vi "FPGAController_v6_Debug.vi"() -> ()   [LabVIEW 2015]
uses:
  Limits_In.ctl
  <vilib>/Utility/miscctls.llb/LVPointTypeDef.ctl
  <vilib>/FPGAPlugInAG/PXIe-7971R/niLvFpga_Open_PXIe-7971R.vi
  <vilib>/Utility/error.llb/Error Cluster From Error Code.vi
  <vilib>/rvi/errors/niLvFpgaAdjustHostInterfaceError.vi
  <userlib>/_OpenG.lib/comparison/comparison.llb/Variant Changed__ogtk.vi
  <vilib>/FPGAPlugInAG/PXIe-7971R/niLvFpga_Close_PXIe-7971R.vi
  <vilib>/rvi/interface/nirviOpenFPGA/nirviOpenFPGA.xnode
  FPGA Bitfiles/FPGA3_FPGATarget_FPGAcode4Test_4n9bj2mwd9A.lvbitx
  <vilib>/rvi/interface/nirviReadWriteControl/nirviReadWriteControl.xnode
  <vilib>/rvi/interface/nirviCloseFPGA/nirviCloseFPGA.xnode
  NiFpgaLv.dll
panel:
  in  "stop":bool
  in  "Tab Control":T1(tab)
  in  "User Trigger?":bool
  in  "User Trigger Distance":fxp<+/-,34,18> format="%.3g"
  in  "Arm/Disarm PSU":bool
  in  "One Shot":bool
  in  "Calibrate":bool
  in  "Threshold Factor":fxp<+/-,32,16>=1.0 format="%.2g"
  out "Limits":T2
  out "Armed":bool
  in  "Clear Points":bool
  in  "Calibration Time (ms)":u32=500
  in  "Boxcar 3 Size Factor":fxp<+/-,32,16>=0.1999969482421875 format="%.2g"
  in  "Charge Error Factor":fxp<+/-,32,16>=1.100006103515625 format="%.2g"
  in  "Max Correlation Factor":fxp<+,32,4>=0.25 format="%.3g"
  out "Latest Particle Stats":T3
  out "Discard Points":i32[][](graph)
  in  "error in (no error)":errorcluster
  out "error out":errorcluster
  out "Runtime Error":errorcluster
  # "User Trigger Distance is\nmeasured in meters from the\nend of the LEIL Chamber\nclosest to the Third Detector"
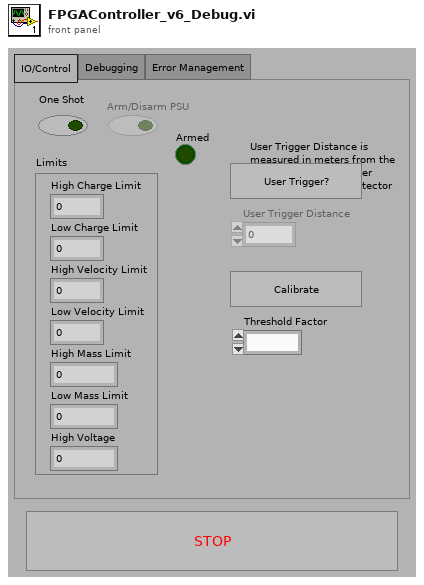
[diagram p1: front panel]
types:
  T1 = enum32{"IO/Control", "Debugging", "Error Management"}
  T2 = typedef "Limits_In.ctl" = cluster{"High Charge Limit":fxp<+,32,-41>, "Low Charge Limit":fxp<+,32,-41>, "High Velocity Limit":fxp<+,18,18>, "Low Velocity Limit":fxp<+,18,18>, "High Mass Limit":fxp<+/-,33,-35>, "Low Mass Limit":fxp<+/-,33,-35>, "High Voltage":fxp<+,16,22>}
  T3 = cluster{"Charge":dbl, "Mass":dbl, "Velocity":i32}
  T4 = enum8{"Enabled", "Disabled", "Disabled and Grayed Out"}
  T5 = typedef "LVPointTypeDef.ctl" = cluster{"Horizontal":i16, "Vertical":i16}
  T6 = cluster{"[0]":fxp<+/-,64,-10>, "[1]":fxp<+/-,64,-10>, "[2]":fxp<+/-,64,-10>, "[3]":fxp<+/-,64,-10>, "[4]":fxp<+/-,64,-10>, "[5]":fxp<+/-,64,-10>, "[6]":fxp<+/-,64,-10>, "[7]":fxp<+/-,64,-10>, "[8]":fxp<+/-,64,-10>, "[9]":fxp<+/-,64,-10>, "[10]":fxp<+/-,64,-10>}
  T7 = cluster{"[0]":fxp<+/-,64,-2>, "[1]":fxp<+/-,64,-2>, "[2]":fxp<+/-,64,-2>, "[3]":fxp<+/-,64,-2>, "[4]":fxp<+/-,64,-2>, "[5]":fxp<+/-,64,-2>, "[6]":fxp<+/-,64,-2>, "[7]":fxp<+/-,64,-2>, "[8]":fxp<+/-,64,-2>, "[9]":fxp<+/-,64,-2>, "[10]":fxp<+/-,64,-2>}
  T8 = cluster{"[0]":i32, "[1]":i32, "[2]":i32, "[3]":i32, "[4]":i32, "[5]":i32, "[6]":i32, "[7]":i32, "[8]":i32, "[9]":i32, "[10]":i32}
  T9 = cluster{"Discard Points 1":cluster{"1":i32, "2":i32, "3":i32, "4":i32, "5":i32, "6":i32, "7":i32, "8":i32, "9":i32, "10":i32, "11":i32}, "Discard Points 2":cluster{"1":i32, "2":i32, "3":i32, "4":i32, "5":i32, "6":i32, "7":i32, "8":i32, "9":i32, "10":i32, "11":i32}, "Discard Points 3":cluster{"1":i32, "2":i32, "3":i32, "4":i32, "5":i32, "6":i32, "7":i32, "8":i32, "9":i32, "10":i32, "11":i32}, "Discard Points 4":cluster{"1":i32, "2":i32, "3":i32, "4":i32, "5":i32, "6":i32, "7":i32, "8":i32, "9":i32, "10":i32, "11":i32}, "Discard Points 5":cluster{"1":i32, "2":i32, "3":i32, "4":i32, "5":i32, "6":i32, "7":i32, "8":i32, "9":i32, "10":i32, "11":i32}, "Discard Points 6":cluster{"1":i32, "2":i32, "3":i32, "4":i32, "5":i32, "6":i32, "7":i32, "8":i32, "9":i32, "10":i32, "11":i32}, "Discard Points 7":cluster{"1":i32, "2":i32, "3":i32, "4":i32, "5":i32, "6":i32, "7":i32, "8":i32, "9":i32, "10":i32, "11":i32}, "Discard Points 8":cluster{"1":i32, "2":i32, "3":i32, "4":i32, "5":i32, "6":i32, "7":i32, "8":i32, "9":i32, "10":i32, "11":i32}, "Discard Points 9":cluster{"1":i32, "2":i32, "3":i32, "4":i32, "5":i32, "6":i32, "7":i32, "8":i32, "9":i32, "10":i32, "11":i32}, "Discard Points 10":cluster{"1":i32, "2":i32, "3":i32, "4":i32, "5":i32, "6":i32, "7":i32, "8":i32, "9":i32, "10":i32, "11":i32}, "Discard Points 11":cluster{"1":i32, "2":i32, "3":i32, "4":i32, "5":i32, "6":i32, "7":i32, "8":i32, "9":i32, "10":i32, "11":i32}}
  T10 = cluster{"1":i32, "2":i32, "3":i32, "4":i32, "5":i32, "6":i32, "7":i32, "8":i32, "9":i32, "10":i32, "11":i32}[]
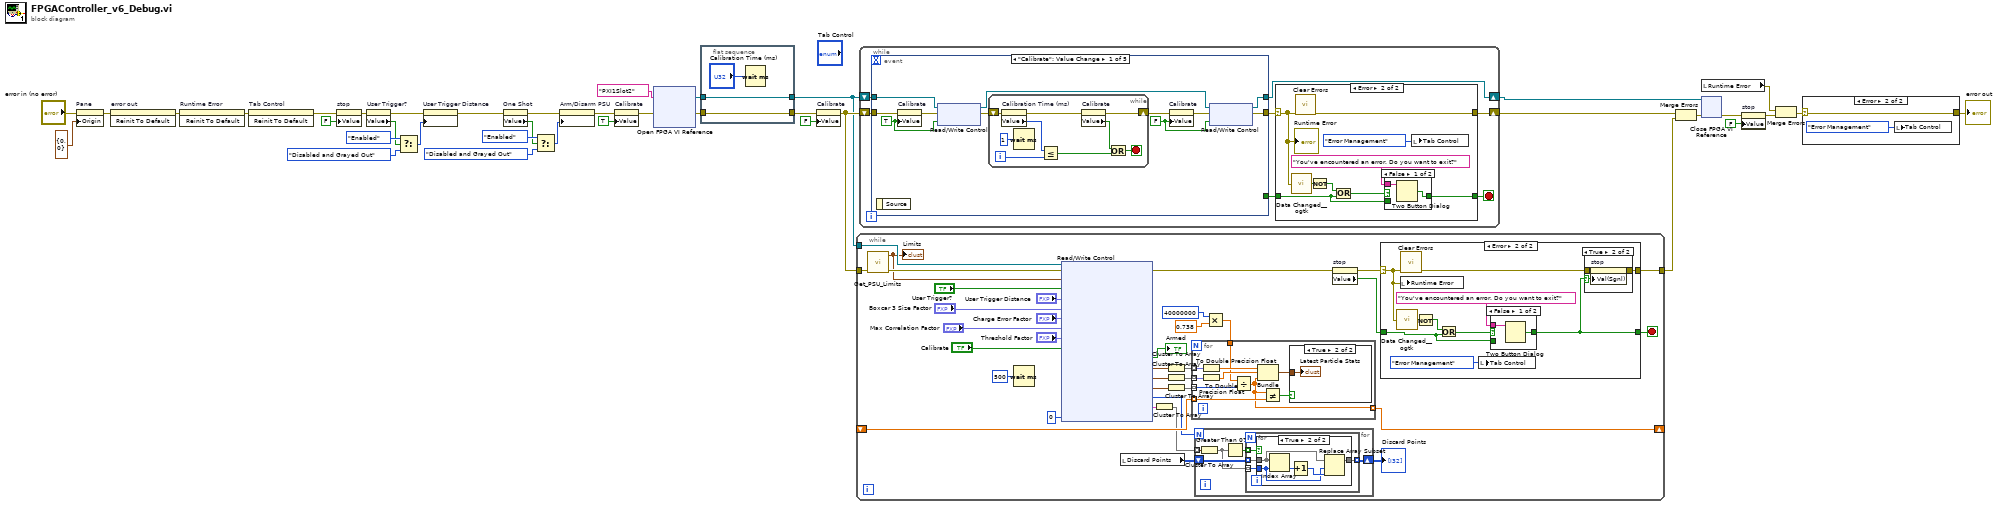
[diagram p0: block diagram]
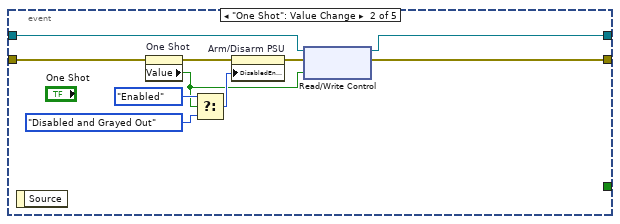
[diagram p10: hidden frame]
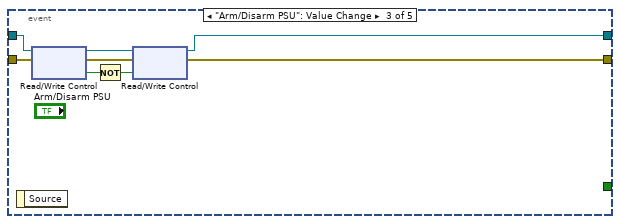
[diagram p11: hidden frame]
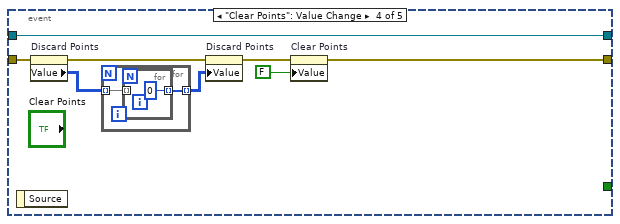
[diagram p12: hidden frame]
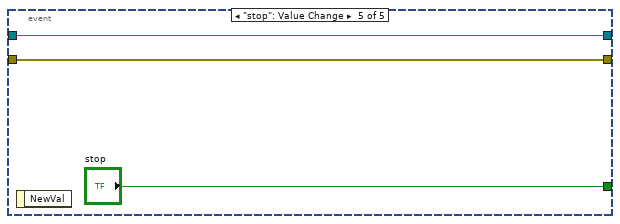
[diagram p13: hidden frame]
diagram:
  n1 = property on="Pane" class="Pane"(error in="error in (no error)", "Origin"=T5 {"Horizontal"=0, "Vertical"=0}) -> (error out=w17:errorcluster)  [unwired: 1 in, 1 out]
  n2 = invoke on="error out" class="Clust (strict)" method="Reinit To Default"(error in=w17) -> (error out=w18:errorcluster)  [unwired: 2 in, 2 out]
  n3 = invoke on="Runtime Error" class="Clust (strict)" method="Reinit To Default"(error in=w18) -> (error out=w16:errorcluster)  [unwired: 2 in, 2 out]
  n4 = invoke on="Tab Control" class="TabCtl (strict)" method="Reinit To Default"(error in=w16) -> (error out=w15:errorcluster)  [unwired: 2 in, 2 out]
  n5 = property on="stop" class="Bool (strict)"(error in=w15, "Value"=FALSE ("stop")) -> (error out=w10:errorcluster)  [unwired: 1 in, 1 out]
  n6 = property on="User Trigger?" class="Bool (strict)"(error in=w10) -> (error out=w20:errorcluster, "Value"=w11:bool)  [unwired: 1 in, 1 out]
  n7 = Select(t=T4."Enabled" ("Disabled"), s=w11, f=T4."Disabled and Grayed Out" ("Disabled")) -> (s? t:f=w22:T4)
  n8 = property on="User Trigger Distance" class="DigNum (strict)"(error in=w20, "DisabledEnum"=w22) -> (error out=w9:errorcluster)  [unwired: 1 in, 1 out]
  n9 = property on="One Shot" class="Bool (strict)"(error in=w9) -> (error out=w29:errorcluster, "Value"=w12:bool)  [unwired: 1 in, 1 out]
  n10 = Select(t=T4."Enabled" ("Disabled"), s=w12, f=T4."Disabled and Grayed Out" ("Disabled")) -> (s? t:f=w23:T4)
  n11 = property on="Arm/Disarm PSU" class="Bool"(error in=w29, "DisabledEnum"=w23) -> (error out=w8:errorcluster)  [unwired: 1 in, 1 out]
  n12 = property on="Calibrate" class="Bool (strict)"(error in=w8, "Value"=TRUE ("One Shot")) -> (error out=w13:errorcluster)  [unwired: 1 in, 1 out]
  n13 = xnode "Open FPGA VI Reference"("error in"=w13, "resource name"=tag "PXI1Slot2") -> ("FPGA VI Reference Out"=w27:refnum<k20>, "error out"=w1:errorcluster)
  n14 = flat-sequence {
    tunnel: [w41] -> w3
    tunnel: w27 -> [w41]
    tunnel: [w40] -> w2
    tunnel: w1 -> [w40]
    frame #0 {
      n15 = Wait (ms)(milliseconds to wait="Calibration Time (ms)") -> ()  [unwired: 1 out]
    }
  }
  n16 = property on="Calibrate" class="Bool (strict)"(error in=w2, "Value"=FALSE ("One Shot")) -> (error out=w6:errorcluster)  [unwired: 1 in, 1 out]
  n17 = while {
    tunnel: [w74] -> w4
    tunnel: w6 -> [w72]
    tunnel: w3 -> [w73]
    shift-right: [w54] -> _
    shift-left: _ -> [w53]
    stop <- w77 stop-if-true
    n18 = call "Get_PSU_Limits.vi"("error in (no error)"=w72) -> ("error out"=w71:errorcluster, "Limits"=w70:T2)  [unwired: 9 in]
    "Limits" <- w70
    n19 = Wait (ms)(milliseconds to wait=u32 500) -> ()  [unwired: 1 out]
    n20 = xnode "Read/Write Control"("FPGA VI Reference In"=w73, "error in"=w71, "Limits"=w70, "User Trigger?"="User Trigger?", "User Trigger Distance"="User Trigger Distance", "Boxcar 3 Size Factor"="Boxcar 3 Size Factor", "Charge Error Factor"="Charge Error Factor", "Max Correlation Factor"="Max Correlation Factor", "Threshold Factor"="Threshold Factor", "Calibrate"="Calibrate", "Particles Discarded"=i16 0) -> ("error out"=w47:errorcluster, "Armed"=→"Armed":bool, "Charge"=w60:T6, "Mass"=w59:T7, "Velocity Count"=w58:T8, "Particles Discarded"=w52:i16, "All Discard Points"=w44:T9)  [unwired: 1 out]
    n21 = local read "Discard Points"() -> (w46:i32[][])
    n22 = Cluster To Array(cluster=w44) -> (array=w51:T10)
    n23 = Cluster To Array(cluster=w60) -> (array=w57:fxp<+/-,64,-10>[])
    n24 = Cluster To Array(cluster=w59) -> (array=w56:fxp<+/-,64,-2>[])
    n25 = Cluster To Array(cluster=w58) -> (array=w55:i32[])
    n26 = for {
      N: w52 -> [_]
      tunnel: w51 -> [w82] mode=indexing
      shift-right: [w78] -> w45
      shift-left: w46 -> [w81]
      n27 = Cluster To Array(cluster=w82) -> (array=w79:i32[])
      n28 = Greater Than 0?(x=w79) -> (x > 0?=w80:bool[])
      n29 = for {
        tunnel: w81 -> [w86] mode=indexing
        tunnel: w79 -> [w85] mode=indexing
        tunnel: w80 -> [w84] mode=indexing
        tunnel: [w83] -> w78 mode=indexing
        n30 = case shown="True" w84 {
          tunnel: w86 -> [w87 w90]
          tunnel: w85 -> [_ w89]
          tunnel: [w87 w88] -> w83
          frame False {
          }
          frame True {
            n31 = Index Array(array=w90, index=w89) -> (element=w92:i32)
            n32 = Increment(x=w92) -> (x+1=w91:i32)
            n33 = Replace Array Subset(array=w90, new element=w91, index=w89) -> (w88:i32[])
          }
        }
      }
    }
    "Discard Points" <- w45
    n34 = Multiply(x=40000000, y=0.738) -> (x*y=w48:dbl)
    n35 = for {
      tunnel: w57 -> [w102] mode=indexing
      tunnel: w56 -> [w101] mode=indexing
      tunnel: w55 -> [w95] mode=indexing
      tunnel: [w93] -> w54 mode=indexing
      tunnel: w53 -> [w94] mode=indexing
      tunnel: w48 -> [w96]
      n36 = To Double Precision Float(number=w102) -> (double precision float=w100:dbl)
      n37 = To Double Precision Float(number=w101) -> (double precision float=w99:dbl)
      n38 = Divide(x=w96, y=w95) -> (x/y=w93:dbl)
      n39 = Bundle(w100, w99, w93) -> (w97:cluster{dbl, dbl, dbl})  [unwired: 1 in]
      n40 = Not Equal?(x=w93, y=w94) -> (x != y?=w98:bool)
      n41 = case shown="True" w98 {
        tunnel: w97 -> [_ w103]
        frame False {
        }
        frame True {
          "Latest Particle Stats" <- w103
        }
      }
    }
    n42 = property on="stop" class="Bool (strict)"(error in=w47) -> (error out=w76:errorcluster, "Value"=w75:bool)  [unwired: 1 in, 1 out]
    n43 = case shown="Error" w76 {
      selector: w76 -> [w105 w110]
      tunnel: [w105 w109] -> w74
      tunnel: [w104 w107] -> w77
      tunnel: w75 -> [w104 w111]
      frame No Error {
      }
      frame Error {
        n44 = call-poly <userlib>:"Data Changed__ogtk.vi"("Variant"=w110) -> ("Changed"=w113:bool)
        n45 = local write "Runtime Error"(w110) -> ()
        n46 = call <vilib>:"Clear Errors.vi"("error in (no error)"=w110) -> ("error out"=w108:errorcluster)  [unwired: 5 in, 1 out]
        n47 = Not(x=w113) -> (.not. x?=w112:bool)
        n48 = Or(x=w112, y=w111) -> (x .or. y?=w114:bool)
        n49 = local write "Tab Control"(T1."Error Management" ("Tab Control")) -> ()
        n50 = case shown="False" w114 {
          tunnel: "You've encountered an error. Do you want to exit?" ("message") -> [w121 _]
          tunnel: [w120 w122] -> w107
          tunnel: w111 -> [_ w122]
          frame False {
            n51 = Two Button Dialog(message=w121) -> (T button?=w120:bool)  [unwired: 2 in]
          }
          frame True {
          }
        }
        n52 = case shown="True" w107 {
          selector: w107 -> [_ w117]
          tunnel: [w116 w119] -> w109
          tunnel: w108 -> [w116 w118]
          frame False {
          }
          frame True {
            n53 = property on="stop" class="Bool (strict)"(error in=w118, "Val(Sgnl)"=w117) -> (error out=w119:errorcluster)  [unwired: 1 in, 1 out]
          }
        }
      }
    }
  }
  n54 = while {
    shift-right: [w123] -> w36
    shift-left: w6 -> [w129]
    shift-right: [w127] -> w37
    shift-left: w3 -> [w128]
    stop <- w125 stop-if-true
    n55 = event shown="[0] \"Calibrate\": Value Change" {
      selector: _ -> [_ _ _ _ _]
      dyn-events: _ -> [_ _ _ _ _]
      timeout: _ -> [_ _ _ _ _]
      tunnel: [_ _ _ _ "stop"] -> w124
      tunnel: w129 -> [w154 w170 w179 w188 w194]
      tunnel: [w146 w165 w181 w182 w194] -> w126
      tunnel: w128 -> [w152 w167 w178 w189 w193]
      tunnel: [w145 w166 w180 w189 w193] -> w127
      event "Calibrate": Value Change {
        w144 = TRUE ("One Shot")
        w148 = FALSE ("One Shot")
        n56 = event-data() -> ()  [unwired: 1 in, 1 out]
        n57 = property on="Calibrate" class="Bool (strict)"(error in=w154, "Value"=w144) -> (error out=w153:errorcluster)  [unwired: 1 in, 1 out]
        n58 = xnode "Read/Write Control"("FPGA VI Reference In"=w152, "error in"=w153, "Calibrate"=w144) -> ("FPGA VI Reference Out"=w147:refnum<k20>, "error out"=w150:errorcluster)
        n59 = while {
          shift-right: [w158] -> w151
          shift-left: w150 -> [w163]
          i -> [w160]
          stop <- w156 stop-if-true
          n60 = property on="Calibration Time (ms)" class="DigNum (strict)"(error in=w163) -> (error out=w157:errorcluster, "Value"=w161:u32)  [unwired: 1 in, 1 out]
          n61 = Wait (ms)(milliseconds to wait=u32 1) -> ()  [unwired: 1 out]
          n62 = Less Or Equal?(x=w161, y=w160) -> (x <= y?=w159:bool)
          n63 = property on="Calibrate" class="Bool (strict)"(error in=w157) -> (error out=w158:errorcluster, "Value"=w155:bool)  [unwired: 1 in, 1 out]
          n64 = Or(x=w155, y=w159) -> (x .or. y?=w156:bool)
        }
        n65 = property on="Calibrate" class="Bool (strict)"(error in=w151, "Value"=w148) -> (error out=w149:errorcluster)  [unwired: 1 in, 1 out]
        n66 = xnode "Read/Write Control"("FPGA VI Reference In"=w147, "error in"=w149, "Calibrate"=w148) -> ("FPGA VI Reference Out"=w145:refnum<k20>, "error out"=w146:errorcluster)
      }
      event "One Shot": Value Change {
        n67 = event-data() -> ()  [unwired: 1 in, 1 out]
        n68 = property on="One Shot" class="Bool (strict)"(error in=w170) -> (error out=w171:errorcluster, "Value"=w164:bool)  [unwired: 1 in, 1 out]
        n69 = Select(t=T4."Enabled" ("Disabled"), s=w164, f=T4."Disabled and Grayed Out" ("Disabled")) -> (s? t:f=w173:T4)
        n70 = property on="Arm/Disarm PSU" class="Bool"(error in=w171, "DisabledEnum"=w173) -> (error out=w168:errorcluster)  [unwired: 1 in, 1 out]
        n71 = xnode "Read/Write Control"("FPGA VI Reference In"=w167, "error in"=w168, "One Shot"=w164) -> ("FPGA VI Reference Out"=w166:refnum<k20>, "error out"=w165:errorcluster)
      }
      event "Arm/Disarm PSU": Value Change {
        n72 = event-data() -> ()  [unwired: 1 in, 1 out]
        n73 = xnode "Read/Write Control"("FPGA VI Reference In"=w178, "error in"=w179) -> ("FPGA VI Reference Out"=w177:refnum<k20>, "error out"=w176:errorcluster, "Armed"=w175:bool)
        n74 = Not(x=w175) -> (.not. x?=w174:bool)
        n75 = xnode "Read/Write Control"("FPGA VI Reference In"=w177, "error in"=w176, "Armed"=w174) -> ("FPGA VI Reference Out"=w180:refnum<k20>, "error out"=w181:errorcluster)
      }
      event "Clear Points": Value Change {
        n76 = event-data() -> ()  [unwired: 1 in, 1 out]
        n77 = property on="Discard Points" class="IntChart (strict)"(error in=w188) -> (error out=w185:errorcluster, "Value"=w187:i32[][])  [unwired: 1 in, 1 out]
        n78 = for {
          tunnel: w187 -> [w191] mode=indexing
          tunnel: [w190] -> w186 mode=indexing
          n79 = for {
            tunnel: w191 -> [_] mode=indexing
            tunnel: [0] -> w190 mode=indexing
          }
        }
        n80 = property on="Discard Points" class="IntChart (strict)"(error in=w185, "Value"=w186) -> (error out=w184:errorcluster)  [unwired: 1 in, 1 out]
        n81 = property on="Clear Points" class="Bool (strict)"(error in=w184, "Value"=FALSE ("Clear Points")) -> (error out=w182:errorcluster)  [unwired: 1 in, 1 out]
      }
      event "stop": Value Change {
        n82 = event-data() -> ()  [unwired: 1 in, 1 out]
      }
    }
    n83 = case shown="Error" w126 {
      selector: w126 -> [w131 w137]
      tunnel: [w131 w140] -> w123
      tunnel: [w130 w138] -> w125
      tunnel: w124 -> [w130 w133]
      frame No Error {
      }
      frame Error {
        n84 = call-poly <userlib>:"Data Changed__ogtk.vi"("Variant"=w137) -> ("Changed"=w135:bool)
        n85 = call <vilib>:"Clear Errors.vi"("error in (no error)"=w137) -> ("error out"=w140:errorcluster)  [unwired: 5 in, 1 out]
        n86 = Not(x=w135) -> (.not. x?=w134:bool)
        n87 = Or(x=w134, y=w133) -> (x .or. y?=w136:bool)
        n88 = case shown="False" w136 {
          tunnel: "You've encountered an error. Do you want to exit?" ("message") -> [w142 _]
          tunnel: [w141 w143] -> w138
          tunnel: w133 -> [_ w143]
          frame False {
            n89 = Two Button Dialog(message=w142) -> (T button?=w141:bool)  [unwired: 2 in]
          }
          frame True {
          }
        }
        n90 = local write "Tab Control"(T1."Error Management" ("Tab Control")) -> ()
        "Runtime Error" <- w137
      }
    }
  }
  n91 = Merge Errors(w36, w4) -> (w5:errorcluster)
  n92 = local read "Runtime Error"() -> (w7:errorcluster)
  n93 = xnode "Close FPGA VI Reference"("FPGA VI Reference In"=w37, "error in"=w5) -> ("error out"=w33:errorcluster)
  n94 = property on="stop" class="Bool (strict)"(error in=w33, "Value"=FALSE ("stop")) -> (error out=w32:errorcluster)  [unwired: 1 in, 1 out]
  n95 = Merge Errors(w7, w32) -> (w30:errorcluster)
  n96 = case shown="Error" w30 {
    selector: w30 -> [w196 w198]
    tunnel: [w196 w198] -> w31
    frame No Error {
    }
    frame Error {
      n97 = local write "Tab Control"(T1."Error Management" ("Tab Control")) -> ()
    }
  }
  "error out" <- w31
